vi "Fan Acceleration Curve J&J.vi"() -> ()   [LabVIEW 2015]
uses:
  <vilib>/Platform/TimedLoop/XDataNode/timing_clust.ctl
  <vilib>/Platform/TimedLoop/XDataNode/nitl_modes.ctl
  <vilib>/Platform/TimedLoop/XDataNode/wakeup.ctl
  <vilib>/platform/TimedLoop/XDataNode/XDataNode.xnode
  <vilib>/Platform/TimedLoop/XDataNode/XDNodeRunTimeDep.lvlib
panel:
  out "error out":errorcluster
  in  "Voltage":dbl
  in  "stop 2":bool
  out "Countrate":cluster{i32[], i32[]}(graph)
  in  "Controls":T1
  in  "stop":bool
  out "counts per Time Increment":dbl(knob) scale=0.0..100.0
  out "output cluster":cluster{i32, dbl}
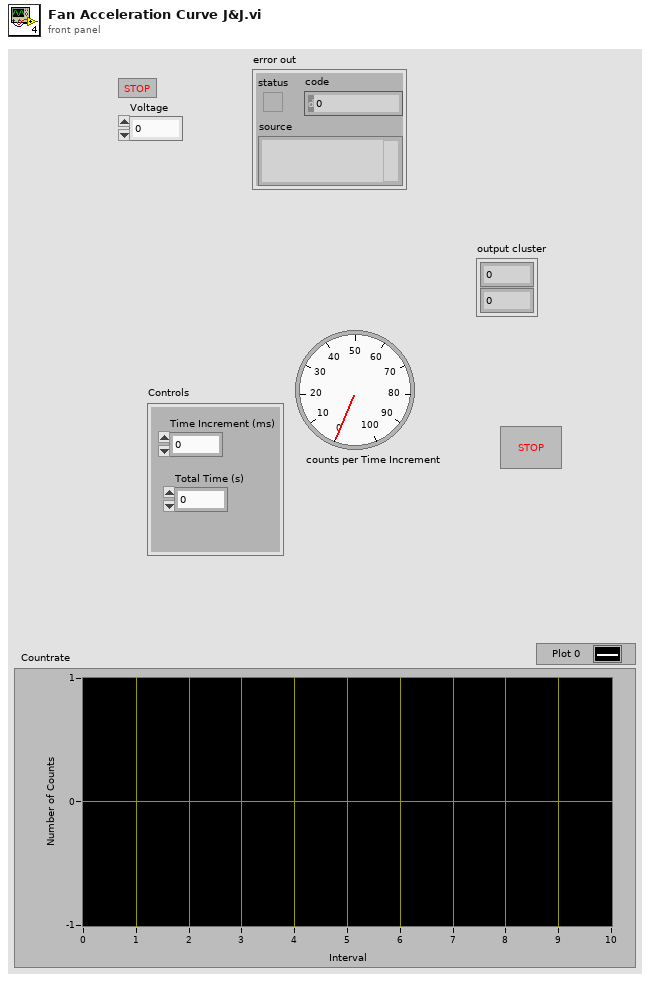
[diagram p1: front panel]
types:
  T1 = cluster{"Time Increment (ms)":i64, "Total Time (s)":dbl}
  T2 = enum16{"open", "replace", "create", "open or create", "replace or create", "replace or create with confirmation"}
  T3 = typedef "XDNodeRunTimeDep.lvlib/timing_clust.ctl" = cluster{"Expected End [f-1]":u64, "Actual End [f-1]":u64, "Finished Late? [f-1]":bool, "Expected End [i-1]":u64, "Actual End [i-1]":u64, "Finished Late? [i-1]":bool, "Expected Start [i]":u64, "Actual Start [i]":u64, "Expected Start [f]":u64, "Actual Start [f]":u64, "Source Name":string, "Structure Name":string, "Period":i64, "Deadline":i64, "Offset":i64, "Start":i64, "Priority":i32, "Timeout":i32, "Mode":T4, "Wakeup Reason":T5, "Error":errorcluster, "Source Type":string, "Secondary Source Type":string, "Global End Time":u64, "Global Start Time":u64, "Frame Duration":u64, "Iteration Duration":u64, "Assigned CPU":i32, "I/O Scan Engine Mode":u32}
  T4 = typedef "XDNodeRunTimeDep.lvlib/nitl_modes.ctl" = enum32{"No Change", "Process missed periods, maintain original phase", "Discard missed periods, maintain original phase", "Process missed periods, ignore original phase", "Discard missed periods, ignore original phase"}
  T5 = typedef "XDNodeRunTimeDep.lvlib/wakeup.ctl" = enum32{"Normal", "Aborted", "Asynchronous wakeup", "Timing source error", "Timed loop error", "Timeout"}
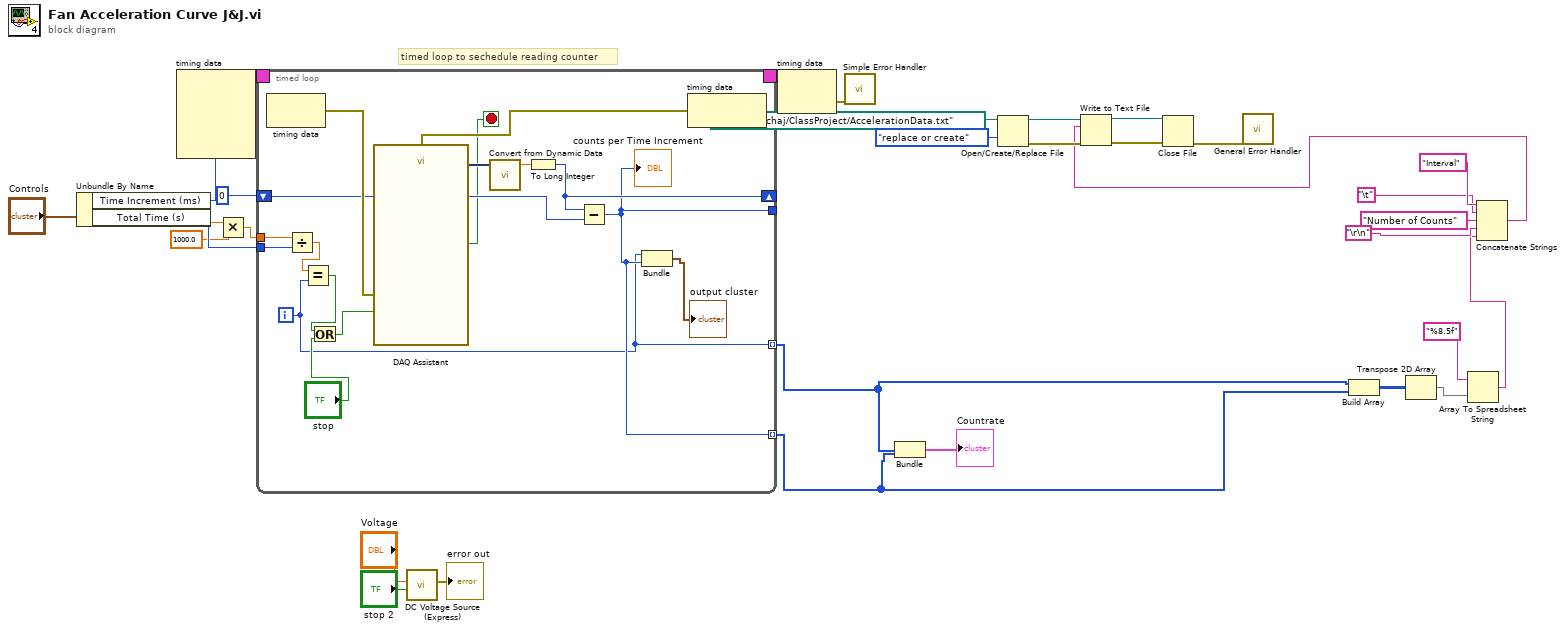
[diagram p0: block diagram]
diagram:
  # "timed loop to sechedule reading counter"
  n1 = Unbundle By Name("Controls") -> ("Time Increment (ms)"=w26:i64, "Total Time (s)"=w25:dbl)
  n2 = node-c288(w26) -> (w31:T3)  [unwired: 3 in]
  n3 = Multiply(x=w25, y=1000.0) -> (x*y=w23:dbl)
  n4 = timed-loop {
    timing: w31 -> [_]
    timing-out: [_] -> w30
    shift-right: [w46] -> _
    shift-left: 0 -> [w42]
    tunnel: [w33] -> _
    tunnel: w26 -> [w41]
    tunnel: w23 -> [w40]
    tunnel: [w33] -> w4 mode=indexing
    tunnel: [w32] -> w5 mode=indexing
    i -> [w32]
    stop <- w39 stop-if-true
    n5 = node-c288() -> (w43:errorcluster)  [unwired: 1 in]
    n6 = Divide(x=w40, y=w41) -> (x/y=w35:dbl)
    n7 = Equal?(x=w35, y=w32) -> (x = y?=w36:bool)
    n8 = Or(x=w36, y="stop") -> (x .or. y?=w37:bool)
    n9 = call "DAQ Assistant"("error in"=w43, "stop (F)"=w37) -> ("data"=w47:dynamicdata, "stopped"=w39:bool, "error out"=w44:errorcluster)  [unwired: 14 in, 1 out]
    n10 = call "Convert from Dynamic Data"("Dynamic Data Type"=w47) -> ("Scalar"=w45:dbl)  [unwired: 3 in]
    n11 = To Long Integer(number=w45) -> (32bit integer=w46:i32)
    n12 = Subtract(x=w46, y=w42) -> (x-y=w33:i32)
    "counts per Time Increment" <- w33
    n13 = Bundle(w32, w33) -> (→"output cluster":cluster{i32, i32})  [unwired: 1 in]
    n14 = node-c288(w44) -> ()  [unwired: 1 out]
  }
  n15 = call "DC Voltage Source (Express).vi"("stop"="stop 2", "Voltage"="Voltage") -> ("error out"=→"error out":errorcluster)  [unwired: 9 in]
  n16 = node-c288(w30) -> (w28:errorcluster)
  n17 = call <vilib>:"Simple Error Handler.vi"("error in (no error)"=w28) -> ()  [unwired: 4 in, 5 out]
  n18 = Bundle(w5, w4) -> (→"Countrate":cluster{i32[], i32[]})  [unwired: 1 in]
  n19 = Open/Create/Replace File(file path (use dialog)=path "C:/Users/atchaj/ClassProject/AccelerationData.txt", operation (0:open)=T2."replace or create") -> (refnum out=w18:refnum<file>, error out=w19:errorcluster)  [unwired: 4 in, 1 out]
  n20 = Build Array(w5, w4) -> (w6:i32[][])
  n21 = Transpose 2D Array(2D array=w6) -> (transposed array=w14:i32[][])
  n22 = Array To Spreadsheet String(array=w14, 3:"%8.5f" ("format string")) -> (spreadsheet string=w9:string)  [unwired: 1 in]
  n23 = Concatenate Strings("Interval" ("string"), "\t", "Number of Counts" ("string"), "\r\n", w9) -> (w8:string)
  n24 = Write to Text File(file (use dialog)=w18, text=w8, error in=w19) -> (refnum out=w17:refnum<file>, error out=w20:errorcluster)  [unwired: 1 in, 1 out]
  n25 = Close File(refnum=w17, error in=w20) -> (error out=w21:errorcluster)  [unwired: 1 out]
  n26 = call <vilib>:"General Error Handler.vi"("error in (no error)"=w21) -> ()  [unwired: 10 in, 5 out]
